vi "WCA_SET_SB_LOCK_POL.vi"(0 "Cartridge Band":u32=10, 1 "Slave Node in":cluster{"Address":i16, "Serial Number":i8[]}={"Address"=19, "Serial Number"=[16, 71, 55, 76, 1, 8, 0, -15]} {"Serial Number" format="%.0x"; "Address" format="%.0x"}, 2 "ObjHandle in":u32, 9 "SET_SB_LOCK_POL":i32, 11 "error in (no error)":errorcluster) -> (4 "ObjHandle out":u32=92930112, 15 "error out":errorcluster)   [LabVIEW 2017]
uses:
  WCA_Global.vi
panel:
  # "Node Address"
  # "Serial Number"
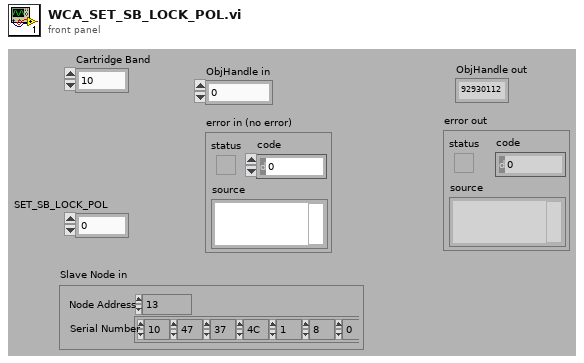
[diagram p1: front panel]
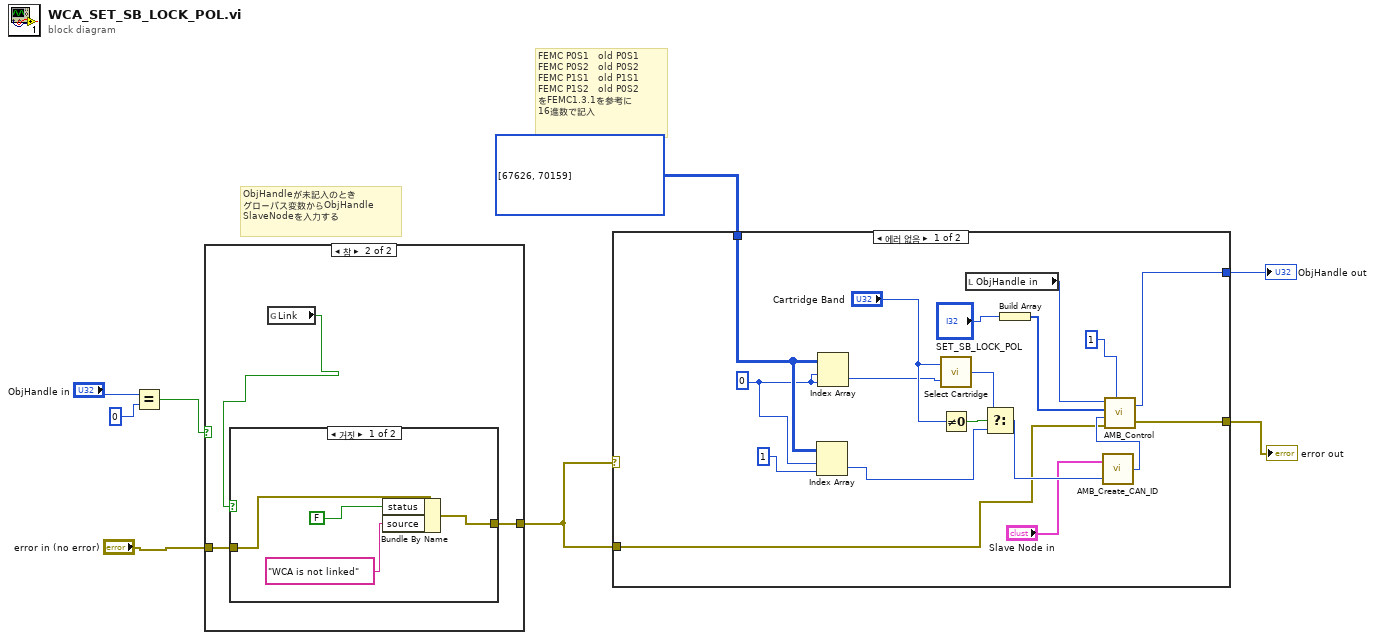
[diagram p0: block diagram]
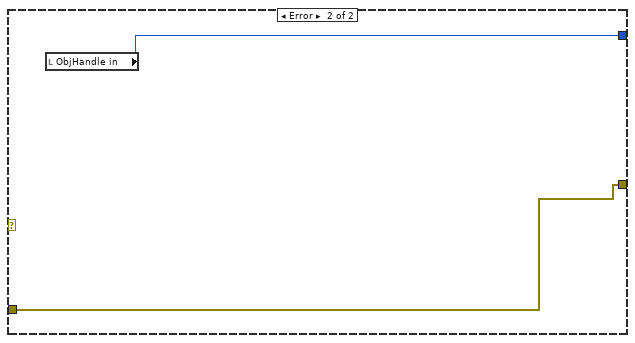
[diagram p2: hidden frame]
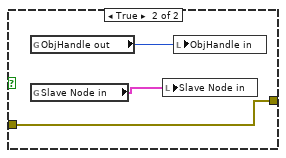
[diagram p4: hidden frame]
diagram:
  # "ObjHandleが未記入のとき\nグローバス変数からObjHandle\nSlaveNodeを入力する"
  # "FEMC P0S1   old P0S1\nFEMC P0S2   old P0S2\nFEMC P1S1   old P1S1\nFEMC P1S2   old P0S2\nをFEMC1.3.1を参考に\n16進数で記入"
  n1 = Equal?(x="ObjHandle in", y=0) -> (x = y?=w6:bool)
  n2 = case shown="참" w6 {
    tunnel: "error in (no error)" -> [w9 w12]
    tunnel: [w9 w11] -> w4
    frame False {
    }
    frame True {
      n3 = global read "WCA_Global.vi" "Link"() -> (w10:bool)
      n4 = case shown="거짓" w10 {
        tunnel: w12 -> [w16 w17]
        tunnel: [w13 w17] -> w11
        frame False {
          n5 = Bundle By Name(cluster=w16, "status"=FALSE, "source"="WCA is not linked") -> (w13:errorcluster)
        }
        frame True {
          n6 = global read "WCA_Global.vi" "ObjHandle out"() -> (w19:u32)
          n7 = global read "WCA_Global.vi" "Slave Node in"() -> (w18:cluster{"Address":i16, "Serial Number":i8[]})
          n8 = local write "Slave Node in"(w18) -> ()
          n9 = local write "ObjHandle in"(w19) -> ()
        }
      }
    }
  }
  n10 = case shown="에러 없음" w4 {
    tunnel: w4 -> [w31 w39]
    tunnel: [w29 w38] -> w3
    tunnel: [w28 w39] -> w2
    tunnel: i32[][] [[67626, 70159]] -> [w25 _]
    frame No Error {
      w20 = 0
      n11 = Index Array(array=w25, index (row)=w20, index (col)=1) -> (element=w26:i32)
      n12 = Index Array(array=w25, index (row)=w20, index (col)=w20) -> (element=w27:i32)
      n13 = call "Select Cartridge.vi"("Relative Address in"=w27, "Cartridge band"="Cartridge Band") -> ("Relative Address out"=w35:u32)
      n14 = Not Equal To 0?(x="Cartridge Band") -> (x != 0?=w36:bool)
      n15 = local read "ObjHandle in"() -> (w30:u32)
      n16 = Select(t=w35, s=w36, f=w26) -> (s? t:f=w34:u32)
      n17 = Build Array("SET_SB_LOCK_POL") -> (w21:i32[])
      n18 = call "AMB_Create_CAN_ID.vi"("Relative Address in"=w34, "Slave Node in"="Slave Node in") -> ("CAN ID out"=w37:u32)
      n19 = call "AMB_Control.vi"("ObjHandle in"=w30, "Data in"=w21, "CAN ID in"=w37, "error in"=w31, "Data Length in"=1) -> ("ObjHandle out"=w29:u32, "error out"=w28:errorcluster)
    }
    frame Error {
      n20 = local read "ObjHandle in"() -> (w38:u32)
    }
  }
  "ObjHandle out" <- w3
  "error out" <- w2
